vi "USBTC08StreamingExample.vi"() -> ()   [LabVIEW 2009]
panel:
  out "Unit Info":T1
  out "handle":i16
  out "error out":errorcluster
  in  "Channel Settings":T2 {"Type # 8" items=["B", "E", "J", "K", "N", "R", "S", "T", "Voltage"]; "Type # 7" items=["B", "E", "J", "K", "N", "R", "S", "T", "Voltage"]; "Type # 6" items=["B", "E", "J", "K", "N", "R", "S", "T", "Voltage"]; "Type # 5" items=["B", "E", "J", "K", "N", "R", "S", "T", "Voltage"]; "Type # 4" items=["B", "E", "J", "K", "N", "R", "S", "T", "Voltage"]; "Type # 3" items=["B", "E", "J", "K", "N", "R", "S", "T", "Voltage"]; "Type # 2" items=["B", "E", "J", "K", "N", "R", "S", "T", "Voltage"]; "Type # 1" items=["B", "E", "J", "K", "N", "R", "S", "T", "Voltage"]}
  out "Overflow":i16[](array[numeric])
  in  "error in (no error)":errorcluster
  in  "Requested No of Samples per channel":i16
  out "minimumIntervalMs":i32
  in  "Mains Frequency":i16(ring) items=["50 Hz", "60 Hz"]
  out "?":dynamicdata(graph)
  in  "Units":enum16{"C°", "F°", "K°", "R°"}(ring)
  in  "stop":bool
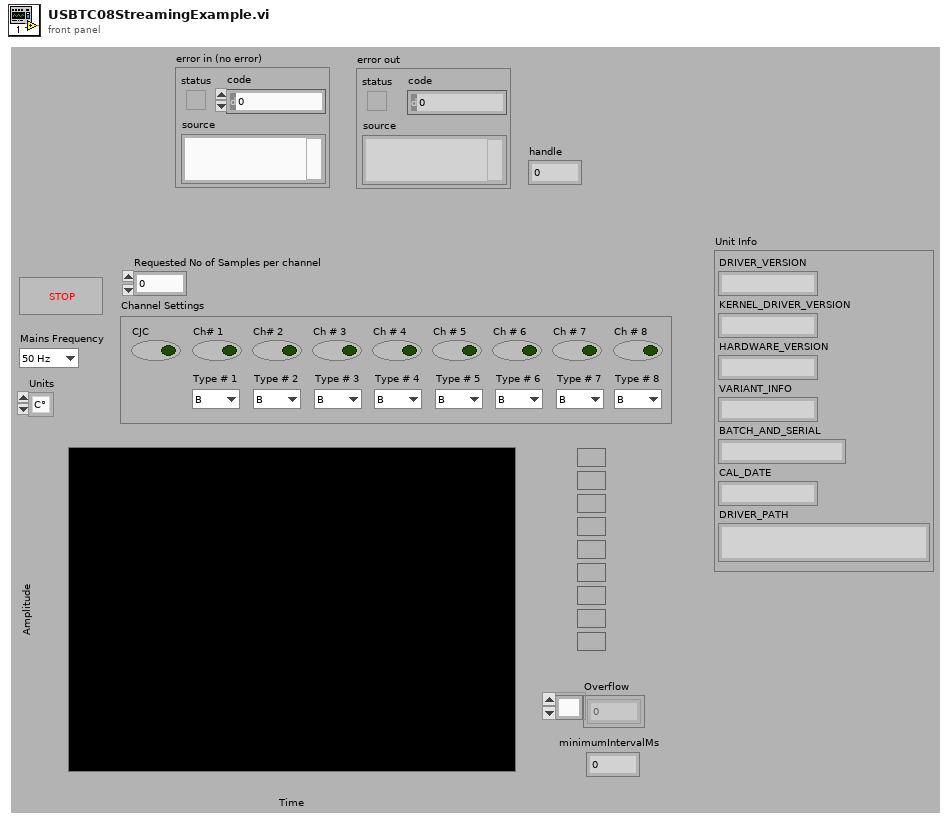
[diagram p1: front panel]
types:
  T1 = cluster{"DRIVER_VERSION":string, "KERNEL_DRIVER_VERSION":string, "HARDWARE_VERSION":string, "VARIANT_INFO":string, "BATCH_AND_SERIAL":string, "CAL_DATE":string, "DRIVER_PATH":string, "[7]":string, "[8]":string, "[9]":string, "[10]":string, "[11]":string, "[12]":string, "[13]":string, "[14]":string}
  T2 = cluster{"Type # 1":i16, "Ch# 1":bool, "Type # 2":i16, "Ch# 2":bool, "Type # 3":i16, "Ch # 3":bool, "Type # 4":i16, "Ch # 4":bool, "Type # 5":i16, "Ch # 5":bool, "Type # 6":i16, "Ch # 6":bool, "Type # 7":i16, "Ch # 7":bool, "Type # 8":i16, "Ch # 8":bool, "CJC":bool}
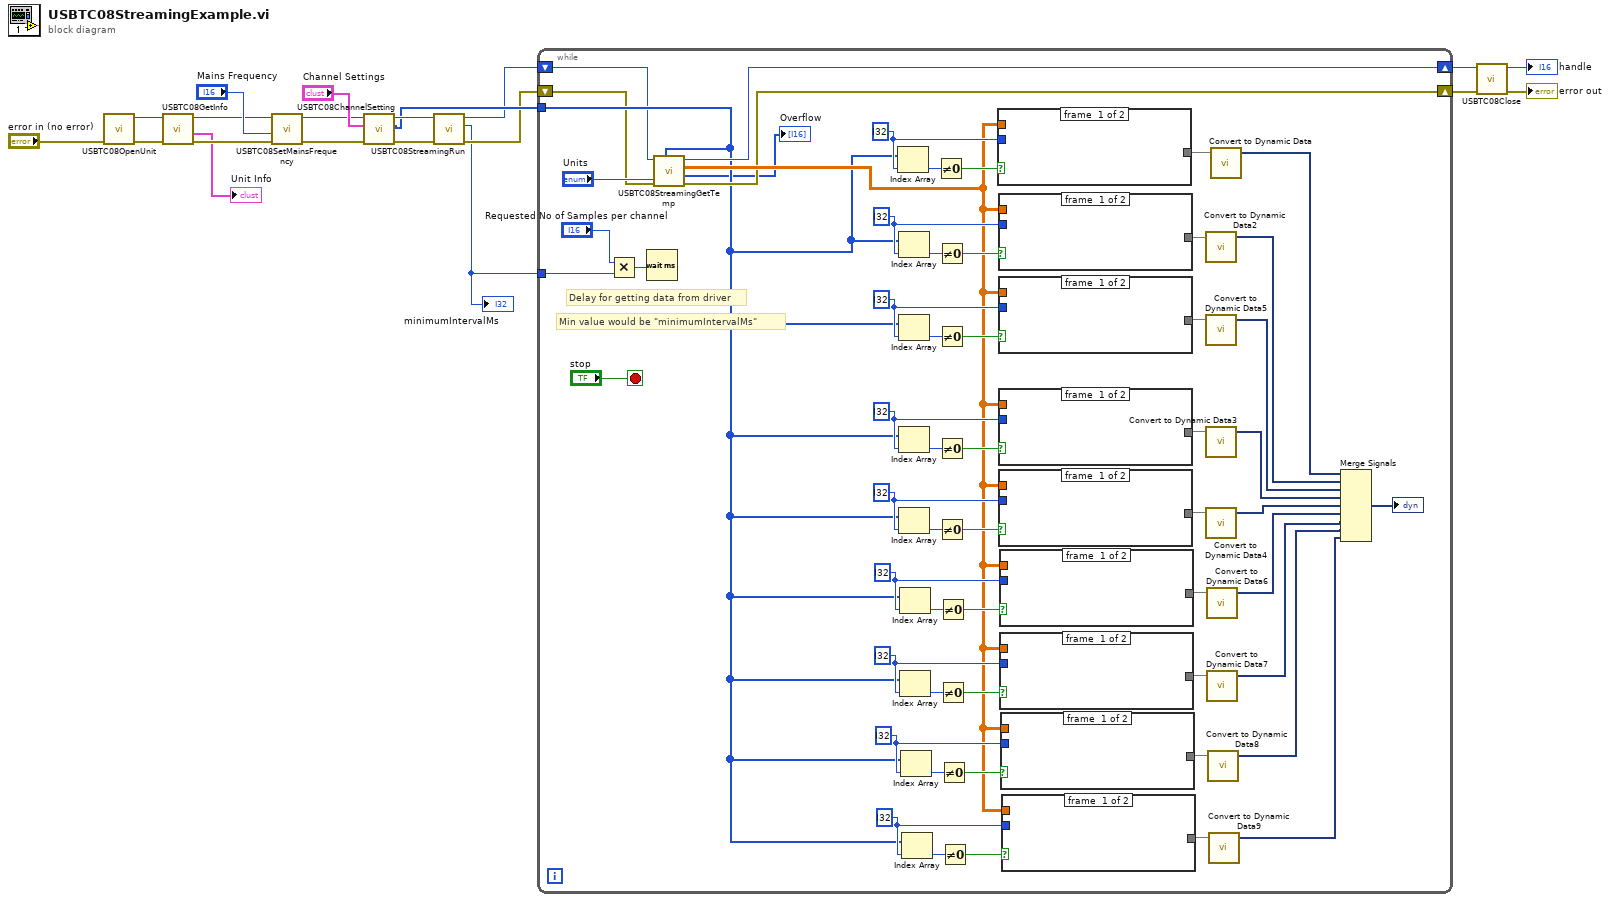
[diagram p0: block diagram]
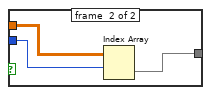
[diagram p2: hidden frame]
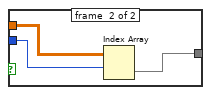
[diagram p3: hidden frame]
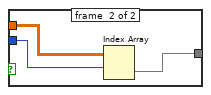
[diagram p4: hidden frame]
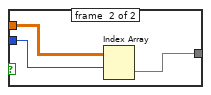
[diagram p5: hidden frame]
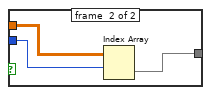
[diagram p6: hidden frame]
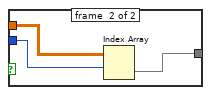
[diagram p7: hidden frame]
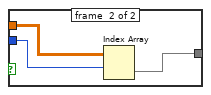
[diagram p8: hidden frame]
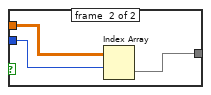
[diagram p9: hidden frame]
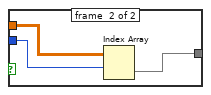
[diagram p10: hidden frame]
diagram:
  n1 = call "USBTC08OpenUnit.vi"("error in (no error)"="error in (no error)") -> ("error out"=w5:errorcluster, "Handle out"=w4:i16)  [unwired: 9 in]
  n2 = call "USBTC08GetInfo.vi"("error in (no error)"=w5, "Handle in"=w4) -> ("error out"=w2:errorcluster, "Unit Info"=→"Unit Info":T1, "Handle out"=w3:i16)  [unwired: 7 in]
  n3 = call "USBTC08SetMainsFrequency.vi"("error in (no error)"=w2, "Mains Frequency"="Mains Frequency", "Handle in"=w3) -> ("error out"=w15:errorcluster, "Handle out"=w16:i16)  [unwired: 7 in]
  n4 = call "USBTC08ChannelSetting.vi"("error in (no error)"=w15, "Channel Settings"="Channel Settings", "Handle In"=w16) -> ("error out"=w18:errorcluster, "Channel Enable Array"=w13:u8[], "Handle out"=w14:i16)  [unwired: 6 in]
  n5 = call "USBTC08StreamingRun.vi"("error in (no error)"=w18, "Handle in"=w14) -> ("error out"=w7:errorcluster, "minimumIntervalMs"=w6:i32, "Handle out"=w8:i16)  [unwired: 7 in]
  "minimumIntervalMs" <- w6
  n6 = while {
    tunnel: w13 -> [w32]
    shift-right: [w78] -> w10
    shift-left: w8 -> [w28]
    shift-right: [w33] -> w9
    shift-left: w7 -> [w29]
    tunnel: w6 -> [w25]
    stop <- "stop" stop-if-true
    w38 = i32 ? ("index (row)")
    w42 = i32 ? ("index (row)")
    w46 = i32 ? ("index (row)")
    w56 = i32 ? ("index (row)")
    w60 = i32 ? ("index (row)")
    w64 = i32 ? ("index (row)")
    w68 = i32 ? ("index (row)")
    w71 = i32 ? ("index (row)")
    w74 = i32 ? ("index (row)")
    # "Min value would be \"minimumIntervalMs\""
    # "Delay for getting data from driver"
    n7 = Multiply(x="Requested No of Samples per channel", y=w25) -> (x*y=w27:i32)
    n8 = Wait (ms)(milliseconds to wait=w27) -> ()  [unwired: 1 out]
    n9 = call "USBTC08StreamingGetTemp.vi"("Units"="Units", "Channel Enable Array"=w32, "error in (no error)"=w29, "Handle in"=w28) -> ("error out"=w33:errorcluster, "Overflow"=→"Overflow":i16[], "Array out"=w36:sgl[][], "Handle out"=w78:i16)  [unwired: 4 in]
    n10 = Index Array(array=w32, index=w74) -> (element=w75:u8)
    n11 = Index Array(array=w32, index=w71) -> (element=w72:u8)
    n12 = Index Array(array=w32, index=w68) -> (element=w69:u8)
    n13 = Index Array(array=w32, index=w64) -> (element=w65:u8)
    n14 = Index Array(array=w32, index=w60) -> (element=w61:u8)
    n15 = Index Array(array=w32, index=w56) -> (element=w57:u8)
    n16 = Index Array(array=w32, index=w46) -> (element=w47:u8)
    n17 = Index Array(array=w32, index=w42) -> (element=w43:u8)
    n18 = Index Array(array=w32, index=w38) -> (element=w39:u8)
    n19 = Not Equal To 0?(x=w75) -> (x != 0?=w76:bool)
    n20 = Not Equal To 0?(x=w72) -> (x != 0?=w73:bool)
    n21 = Not Equal To 0?(x=w69) -> (x != 0?=w70:bool)
    n22 = Not Equal To 0?(x=w65) -> (x != 0?=w66:bool)
    n23 = Not Equal To 0?(x=w61) -> (x != 0?=w62:bool)
    n24 = Not Equal To 0?(x=w57) -> (x != 0?=w58:bool)
    n25 = Not Equal To 0?(x=w47) -> (x != 0?=w48:bool)
    n26 = Not Equal To 0?(x=w43) -> (x != 0?=w44:bool)
    n27 = Not Equal To 0?(x=w39) -> (x != 0?=w40:bool)
    n28 = case shown="True" w76 {
      tunnel: [_ w105] -> w24
      tunnel: w74 -> [_ w104]
      tunnel: w36 -> [_ w103]
      frame #0 {
      }
      frame #1 {
        n29 = Index Array(array=w103, index (row)=w104) -> (element=w105:sgl[])  [unwired: 1 in]
      }
    }
    n30 = case shown="True" w73 {
      tunnel: [_ w102] -> w23
      tunnel: w71 -> [_ w101]
      tunnel: w36 -> [_ w100]
      frame #0 {
      }
      frame #1 {
        n31 = Index Array(array=w100, index (row)=w101) -> (element=w102:sgl[])  [unwired: 1 in]
      }
    }
    n32 = case shown="True" w70 {
      tunnel: [_ w99] -> w67
      tunnel: w68 -> [_ w98]
      tunnel: w36 -> [_ w97]
      frame #0 {
      }
      frame #1 {
        n33 = Index Array(array=w97, index (row)=w98) -> (element=w99:sgl[])  [unwired: 1 in]
      }
    }
    n34 = case shown="True" w66 {
      tunnel: [_ w96] -> w63
      tunnel: w64 -> [_ w95]
      tunnel: w36 -> [_ w94]
      frame #0 {
      }
      frame #1 {
        n35 = Index Array(array=w94, index (row)=w95) -> (element=w96:sgl[])  [unwired: 1 in]
      }
    }
    n36 = case shown="True" w62 {
      tunnel: [_ w93] -> w59
      tunnel: w60 -> [_ w92]
      tunnel: w36 -> [_ w91]
      frame #0 {
      }
      frame #1 {
        n37 = Index Array(array=w91, index (row)=w92) -> (element=w93:sgl[])  [unwired: 1 in]
      }
    }
    n38 = case shown="True" w58 {
      tunnel: [_ w90] -> w55
      tunnel: w56 -> [_ w89]
      tunnel: w36 -> [_ w88]
      frame #0 {
      }
      frame #1 {
        n39 = Index Array(array=w88, index (row)=w89) -> (element=w90:sgl[])  [unwired: 1 in]
      }
    }
    n40 = case shown="True" w48 {
      tunnel: [_ w87] -> w45
      tunnel: w46 -> [_ w86]
      tunnel: w36 -> [_ w85]
      frame #0 {
      }
      frame #1 {
        n41 = Index Array(array=w85, index (row)=w86) -> (element=w87:sgl[])  [unwired: 1 in]
      }
    }
    n42 = case shown="True" w44 {
      tunnel: [_ w84] -> w41
      tunnel: w42 -> [_ w83]
      tunnel: w36 -> [_ w82]
      frame #0 {
      }
      frame #1 {
        n43 = Index Array(array=w82, index (row)=w83) -> (element=w84:sgl[])  [unwired: 1 in]
      }
    }
    n44 = case shown="True" w40 {
      tunnel: [_ w81] -> w37
      tunnel: w38 -> [_ w80]
      tunnel: w36 -> [_ w79]
      frame #0 {
      }
      frame #1 {
        n45 = Index Array(array=w79, index (row)=w80) -> (element=w81:sgl[])  [unwired: 1 in]
      }
    }
    n46 = call "Convert to Dynamic Data2"("Array"=w23) -> ("Dynamic Data Type"=w53:dynamicdata)  [unwired: 3 in]
    n47 = call "Convert to Dynamic Data5"("Array"=w67) -> ("Dynamic Data Type"=w52:dynamicdata)  [unwired: 3 in]
    n48 = call "Convert to Dynamic Data3"("Array"=w63) -> ("Dynamic Data Type"=w51:dynamicdata)  [unwired: 3 in]
    n49 = call "Convert to Dynamic Data4"("Array"=w59) -> ("Dynamic Data Type"=w50:dynamicdata)  [unwired: 3 in]
    n50 = call "Convert to Dynamic Data6"("Array"=w55) -> ("Dynamic Data Type"=w49:dynamicdata)  [unwired: 3 in]
    n51 = call "Convert to Dynamic Data7"("Array"=w45) -> ("Dynamic Data Type"=w35:dynamicdata)  [unwired: 3 in]
    n52 = call "Convert to Dynamic Data8"("Array"=w41) -> ("Dynamic Data Type"=w34:dynamicdata)  [unwired: 3 in]
    n53 = call "Convert to Dynamic Data9"("Array"=w37) -> ("Dynamic Data Type"=w22:dynamicdata)  [unwired: 3 in]
    n54 = call "Convert to Dynamic Data"("Array"=w24) -> ("Dynamic Data Type"=w54:dynamicdata)  [unwired: 3 in]
    n55 = Merge Signals(w54, w53, w52, w51, w50, w49, w35, w34, w22) -> (→"?":dynamicdata)
  }
  n56 = call "USBTC08Close.vi"("error in (no error)"=w9, "Handle in"=w10) -> ("error out"=→"error out":errorcluster, "handle"=→"handle":i16)  [unwired: 8 in]
